vi "Post-Build Action PharLap.vi"(5 "Files Generated by Build":path[](array[path]), 6 "Top Level/Always Included VIs":path[](array[path]), 7 "Destination Path":path, 8 "error in (no error)":errorcluster, 9 "Target Name":string, 10 "Build Specification Name":string, 11 "Project Path":path) -> (0 "error out":errorcluster)   [LabVIEW 2017]
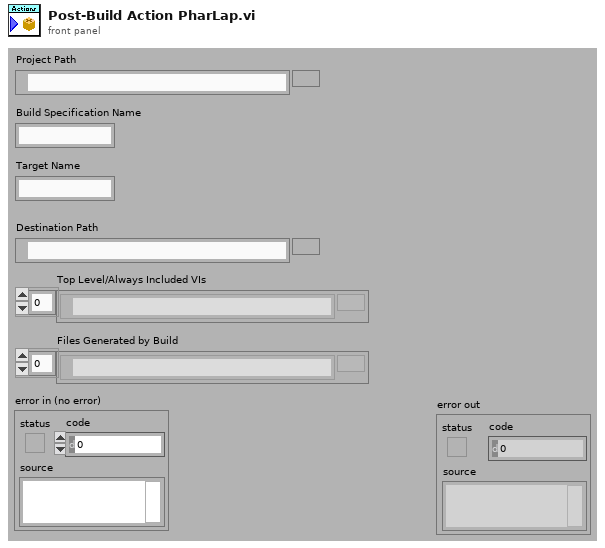
[diagram p1: front panel]
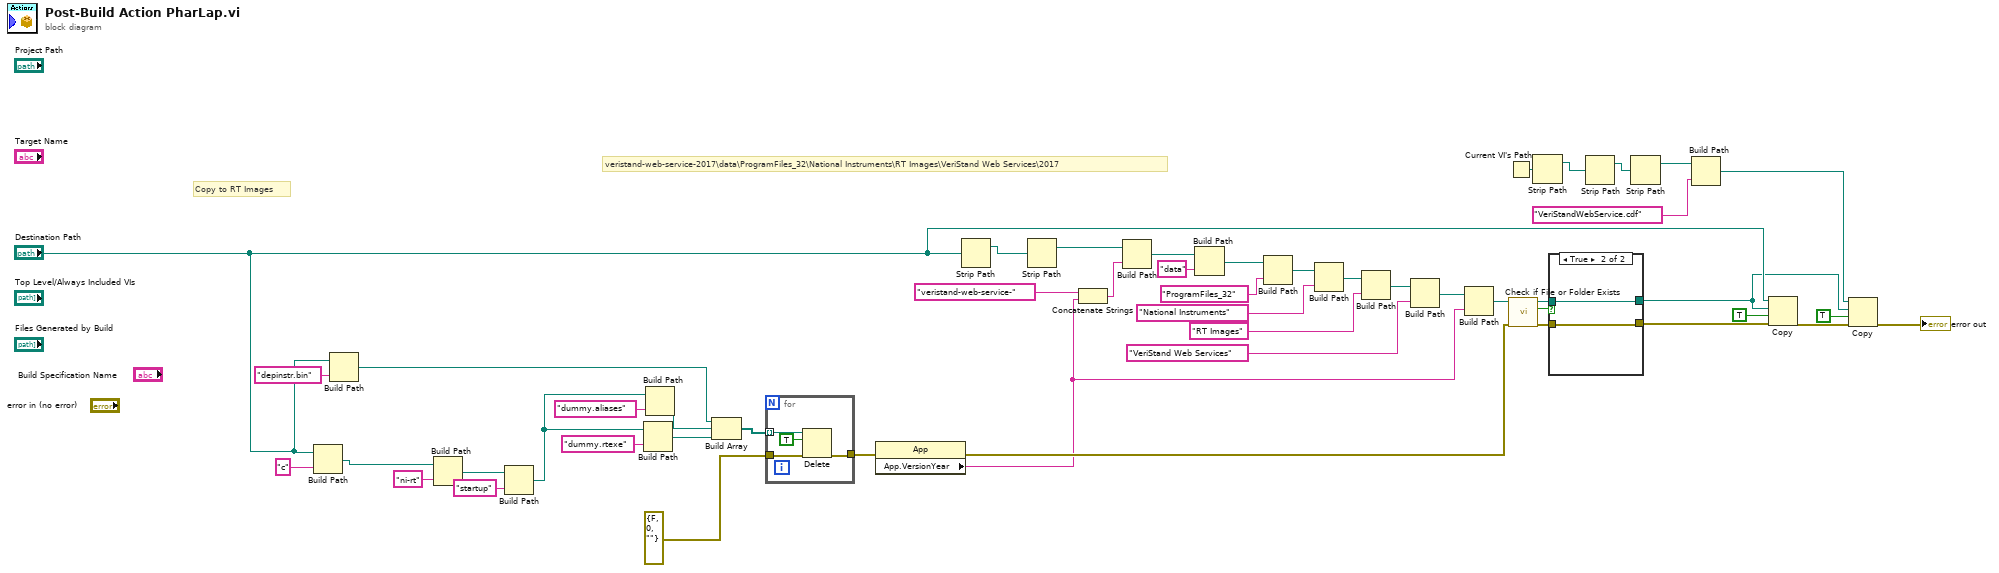
[diagram p0: block diagram]
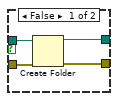
[diagram p2: hidden frame]
diagram:
  # "veristand-web-service-2017\\data\\ProgramFiles_32\\National Instruments\\RT Images\\VeriStand Web Services\\2017"
  # "Copy to RT Images"
  n1 = Build Path(base path="Destination Path", name or relative path="c") -> (appended path=w36:path)
  n2 = Build Path(base path="Destination Path", name or relative path="depinstr.bin") -> (appended path=w34:path)
  n3 = Build Path(base path=w36, name or relative path="ni-rt") -> (appended path=w44:path)
  n4 = Build Path(base path=w44, name or relative path="startup") -> (appended path=w40:path)
  n5 = Build Path(base path=w40, name or relative path="dummy.rtexe") -> (appended path=w38:path)
  n6 = Build Path(base path=w40, name or relative path="dummy.aliases") -> (appended path=w39:path)
  n7 = Build Array(w34, w39, w38) -> (w37:path[])
  n8 = for {
    tunnel: w37 -> [w53] mode=indexing
    tunnel: errorcluster {"status"=FALSE, "code"=0, "source"=""} ("error out") -> [w52]
    tunnel: [w51] -> w30
    n9 = Delete(path (use dialog)=w53, entire hierarchy (F)=TRUE, error in=w52) -> (error out=w51:errorcluster)  [unwired: 2 in, 2 out]
  }
  n10 = property class="App"(error in=w30) -> (error out=w12:errorcluster, "App.VersionYear"=w2:string)  [unwired: 1 in, 1 out]
  n11 = Strip Path(path="Destination Path") -> (stripped path=w5:path)  [unwired: 1 out]
  n12 = Strip Path(path=w5) -> (stripped path=w4:path)  [unwired: 1 out]
  n13 = Concatenate Strings("veristand-web-service-", w2) -> (w29:string)
  n14 = Build Path(base path=w4, name or relative path=w29) -> (appended path=w27:path)
  n15 = Build Path(base path=w27, name or relative path="data") -> (appended path=w25:path)
  n16 = Build Path(base path=w25, name or relative path="ProgramFiles_32") -> (appended path=w23:path)
  n17 = Build Path(base path=w23, name or relative path="National Instruments") -> (appended path=w21:path)
  n18 = Build Path(base path=w21, name or relative path="RT Images") -> (appended path=w19:path)
  n19 = Build Path(base path=w19, name or relative path="VeriStand Web Services") -> (appended path=w17:path)
  n20 = Build Path(base path=w17, name or relative path=w2) -> (appended path=w16:path)
  n21 = Current VI's Path() -> (path=w49:path)
  n22 = call <vilib>:"Check if File or Folder Exists.vi"("error in (no error)"=w12, "path"=w16) -> ("error out"=w13:errorcluster, "file or folder exists?"=w15:bool, "dup path"=w14:path)  [unwired: 7 in]
  n23 = Strip Path(path=w49) -> (stripped path=w48:path)  [unwired: 1 out]
  n24 = case shown="True" w15 {
    tunnel: w14 -> [w57 w58]
    tunnel: w13 -> [w56 w59]
    tunnel: [w55 w59] -> w10
    tunnel: [w54 w58] -> w1
    frame False {
      n25 = Create Folder(path (use dialog)=w57, error in=w56) -> (created path=w54:path, error out=w55:errorcluster)  [unwired: 1 in, 1 out]
    }
    frame True {
    }
  }
  n26 = Strip Path(path=w48) -> (stripped path=w32:path)  [unwired: 1 out]
  n27 = Strip Path(path=w32) -> (stripped path=w31:path)  [unwired: 1 out]
  n28 = Build Path(base path=w31, name or relative path="VeriStandWebService.cdf") -> (appended path=w6:path)
  n29 = Copy(8:w10, 9:TRUE ("overwrite (F)"), 10:w1, 11:"Destination Path") -> (0:w8:errorcluster)  [unwired: 1 in, 2 out]
  n30 = Copy(8:w8, 9:TRUE ("overwrite (F)"), 10:w1, 11:w6) -> (0:→"error out":errorcluster)  [unwired: 1 in, 2 out]
